vi "Read Library_Source_Folder from VIPB.vi"(8 "error in":errorcluster, 10 "VIPB File Path":path) -> (0 "error out":errorcluster, 1 "appended path":path, 2 "Library_Source_Folder":string)   [LabVIEW 2019, in "VIPM.lvlib"]
uses:
  VIPM.lvlib
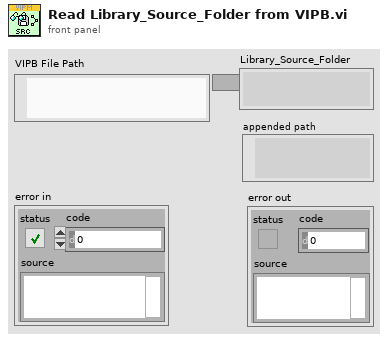
[diagram p1: front panel]
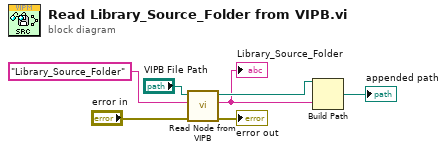
[diagram p0: block diagram]
diagram:
  n1 = call "Read Node from VIPB.vi"("error in (no error)"="error in", "Node Name"="Library_Source_Folder" ("XPath expression"), "VIPB File Path"="VIPB File Path") -> ("error out"=→"error out":errorcluster, "node text"=w1:string, "VIPB File Path out"=w2:path)  [unwired: 6 in]
  "Library_Source_Folder" <- w1
  n2 = Build Path(base path=w2, name or relative path=w1) -> (appended path=→"appended path":path)
